vi "Explain Error.vi"(8 "error in":errorcluster, 10 "Explanation":string) -> (0 "error out":errorcluster)   [LabVIEW 2015]
doc: "If \"Error In\" contains an error, prepend \"Explanation\" to its error documentation."
uses:
  <vilib>/Utility/error.llb/DialogType.ctl
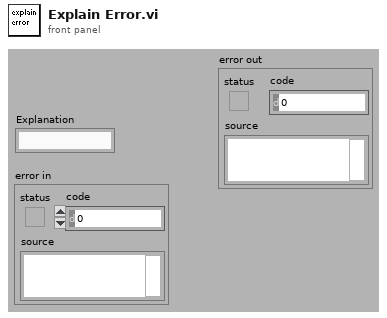
[diagram p1: front panel]
types:
  T1 = typedef "DialogType.ctl" = u16
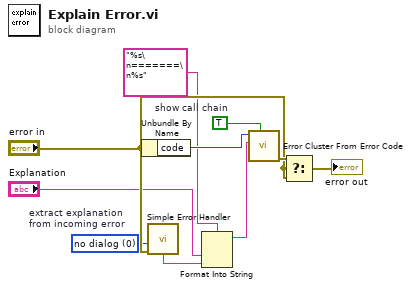
[diagram p0: block diagram]
diagram:
  w1 = TRUE  # show call chain
  w7 = T1 0 items=["no dialog", "OK message", "continue or stop message", "OK message + warnings", "continue/stop + warnings"]  # extract explanation from incoming error
  n1 = Unbundle By Name("error in") -> ("code"=w6:i32)
  n2 = call <vilib>:"Simple Error Handler.vi"("type of dialog (OK msg:1)"=w7, "error in (no error)"="error in") -> ("message"=w2:string)  [unwired: 7 out]
  n3 = Format Into String(format string="%s\n=======\n%s" ("String 2"), "Explanation", w2) -> (resulting string=w9:string)  [unwired: 2 in, 1 out]
  n4 = call <vilib>:"Error Cluster From Error Code.vi"("show call chain? (False)"=w1, "error message (\"\")"=w9, "error code (0)"=w6) -> ("error out"=w10:errorcluster)  [unwired: 1 in, 5 out]
  n5 = Select(t=w10, s="error in", f="error in") -> (s? t:f=→"error out":errorcluster)
